vi "SL_Barcode_Analysis.vi"(11 "Refnum in":T1) -> (1 "BarCode Found?":bool, 2 "Barcode Read":cluster{"Data":string, "Barcode Type":string}[](array[cluster]), 3 "Refnum out":T1(plugin-control))   [LabVIEW 2015]
uses:
  <vilib>/vision/Image Controls.llb/IMAQ Image.ctl
  <vilib>/vision/Instrument.llb/Barcode Search Options.ctl
  <vilib>/vision/NI_Vision_Development_Module.lvlib
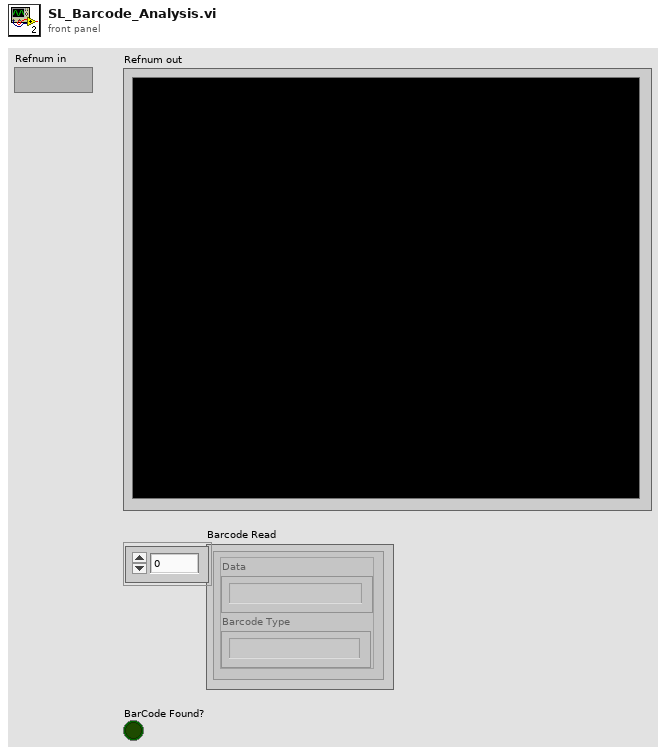
[diagram p1: front panel]
types:
  T1 = typedef "IMAQ Image.ctl" = refnum<image>
  T2 = cluster{"Calculate Grading Report":bool, "Scan Width ":i32}
  T3 = typedef "Barcode Search Options.ctl" = cluster{"Min Bar Width":u32, "Min Edge Strength":u32, "Min Bars":u32, "Skip Location Search?":bool}
  T4 = cluster{"Data":string, "Special Char 1":string, "Special Char 2":string, "Checksum(s)":string, "Barcode Type":u32, "Confidence Level":sgl, "Bounding Box":cluster{"x":sgl, "y":sgl}[]}[]
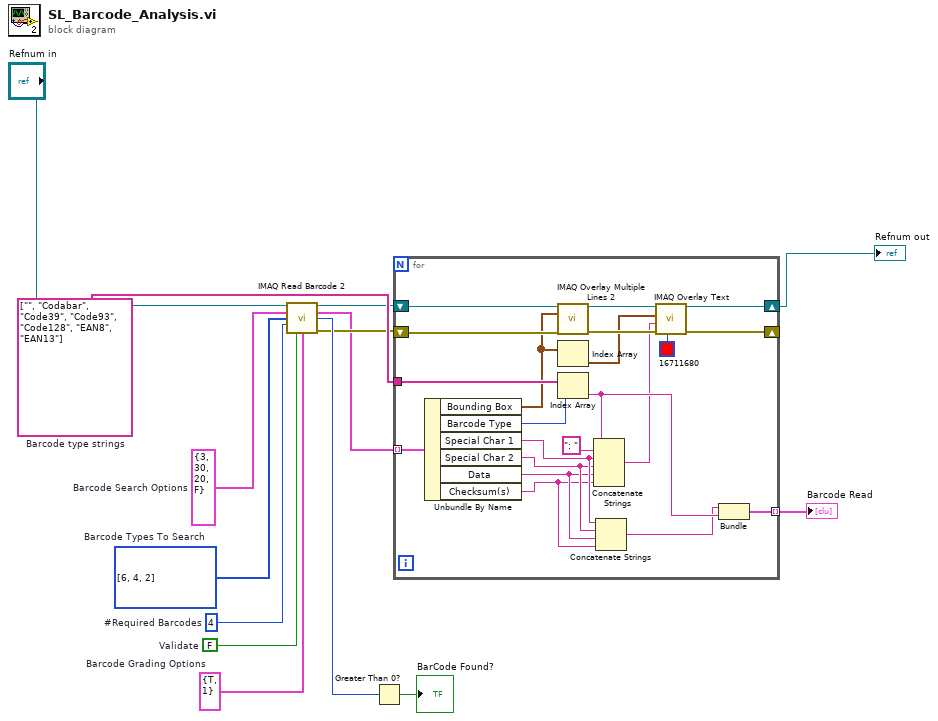
[diagram p0: block diagram]
diagram:
  w12 = string[] ["", "Codabar", "Code39", "Code93", "Code128", "EAN8", "EAN13"]  # Barcode type strings
  w9 = T2 {"Calculate Grading Report"=TRUE, "Scan Width "=1}  # Barcode Grading Options
  w8 = T3 {"Min Bar Width"=3, "Min Edge Strength"=30, "Min Bars"=20, "Skip Location Search?"=FALSE}  # Barcode Search Options
  w1 = u32 4  # #Required Barcodes
  w4 = u32[] [6, 4, 2] items=["Reserved", "Codabar", "Code 39", "Code 93", "Code 128", "EAN 8", "EAN 13", "Interleaved 2 of 5", "MSI", "UPCA", "Pharmacode", "RSS Limited"]  # Barcode Types To Search
  w7 = FALSE  # Validate
  n1 = call "IMAQ Read Barcode 2"("Image"="Refnum in", "Barcode Search Options"=w8, "Barcode Types To Search"=w4, "Num of Required Barcodes"=w1, "Validate"=w7, "Barcode Grading Options"=w9) -> ("Image (duplicate)"=w3:T1, "Barcodes"=w2:T4, "Num of Barcodes"=w13:u32, "error out"=w5:errorcluster)  [unwired: 5 in, 1 out]
  n2 = Greater Than 0?(x=w13) -> (x > 0?=→"BarCode Found?":bool)
  n3 = for {
    tunnel: w2 -> [w35] mode=indexing
    tunnel: w12 -> [w34]
    shift-right: [w30] -> w6
    shift-left: w3 -> [w26]
    shift-right: [w27] -> _
    shift-left: w5 -> [w29]
    tunnel: [w22] -> w10 mode=indexing
    n4 = Unbundle By Name(w35) -> ("Bounding Box"=w25:cluster{"x":sgl, "y":sgl}[], "Barcode Type"=w23:u32, "Special Char 1"=w19:string, "Special Char 2"=w18:string, "Data"=w17:string, "Checksum(s)"=w16:string)
    n5 = call "IMAQ Overlay Multiple Lines 2"("Image"=w26, "Line End Points"=w25, "error in (no error)"=w29) -> ("Image Out"=w32:T1, "error out"=w28:errorcluster)  [unwired: 11 in]
    n6 = Index Array(array=w25) -> (element=w24:cluster{"x":sgl, "y":sgl})  [unwired: 1 in]
    n7 = Index Array(array=w34, index=w23) -> (element=w21:string)
    n8 = Concatenate Strings(w21, ": " ("string"), w19, w18, w17, w16) -> (w20:string)
    n9 = Concatenate Strings(w19, w18, w17, w16) -> (w15:string)
    n10 = call "IMAQ Overlay Text"("Text Color (black)"=u32 16711680, "error in (no error)"=w28, "String"=w20, "Origin"=w24, "Image"=w32) -> ("error out"=w27:errorcluster, "Image Out"=w30:T1)  [unwired: 5 in]
    n11 = Bundle(w15, w21) -> (w22:cluster{string, string})  [unwired: 1 in]
  }
  "Refnum out" <- w6
  "Barcode Read" <- w10
